vi "Read All RADC.vi"() -> ()   [LabVIEW 2013, in "HadCon.lvlib"]
doc: "Example VI reading all ADC raw values."
uses:
  <instrlib>/HadCon/HadCon.lvlib
panel:
  in  "# Channels (F:4)":bool
  out "ADC Raw Values":u32[](array[numeric]) format="%.0x"
  out "Error Out":errorcluster
  in  "VISA resource name":refnum<visa-resource-name>
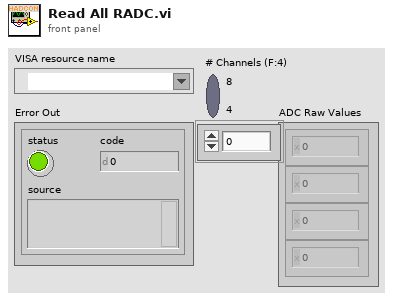
[diagram p1: front panel]
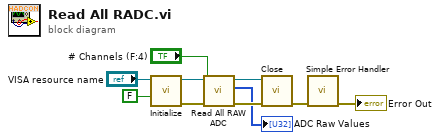
[diagram p0: block diagram]
diagram:
  n1 = call <instrlib>:"Initialize.vi"("Reset (True)"=FALSE, "VISA resource name"="VISA resource name") -> ("error out"=w6:errorcluster, "VISA resource name out"=w7:refnum<visa-resource-name>)  [unwired: 8 in]
  n2 = call <instrlib>:"Read All RAW ADC.vi"("error in (no error)"=w6, "# Channels (F:4)"="# Channels (F:4)", "VISA resource name"=w7) -> ("error out"=w5:errorcluster, "ADC Raw Values"=→"ADC Raw Values":u16[], "VISA resource name out"=w4:refnum<visa-resource-name>)  [unwired: 6 in]
  n3 = call <instrlib>:"Close.vi"("error in (no error)"=w5, "VISA resource name"=w4) -> ("error out"=w10:errorcluster)  [unwired: 9 in]
  n4 = call <vilib>:"Simple Error Handler.vi"("error in (no error)"=w10) -> ("error out"=→"Error Out":errorcluster)  [unwired: 4 in, 4 out]
